vi "Write Identifier Tag.vi"(9 "Array":T3(array[cluster]), 10 "Cluster":T5 {"Main Config"."PR Module Configs"."Settings"."PID 2 Parameters"."output range"."output low" format="%.2f"; "Main Config"."PR Module Configs"."Settings"."PID 2 Parameters"."output range"."output high" min=0.0 max=100.0 format="%.2f"; "Main Config"."PR Module Configs"."Settings"."PID 2 Parameters"."PID gains"."derivative time (Td, min)" format="%.3f"; "Main Config"."PR Module Configs"."Settings"."PID 2 Parameters"."PID gains"."integral time (Ti, min)" format="%.3f"; "Main Config"."PR Module Configs"."Settings"."PID 2 Parameters"."PID gains"."proportional gain (Kc)" format="%.3f"; "Main Config"."Steps"."Control" items=["Pump %", "Setpoint"]; "Main Config"."TCU Module Configs"."Settings"."Huber Unistat 410 Settings"."Address" min=0 max=99 format="%02.0f"; "Main Config"."TCU Module Configs"."Settings"."Julabo FP-50 Settings"."Pump Power" min=0 max=8 step=1; "Main Config"."TCU Module Configs"."Settings"."Lauda Settings"."Pump Power" min=0 max=8 step=1; "Main Config"."Flow Module Configs"."Settings"."Bronkhorst M14 Settings"."Smoothing Steps" min=1 step=1; "Main Config"."Flow Module Configs"."Settings"."Bronkhorst M13 Settings"."Smoothing Steps" min=1 step=1; "Main Config"."Pump Module Configs"."Settings"."Ismatech 3 Channel Settings"."Channel Number" min=0 max=3; "Main Config"."Pump Module Configs"."Settings"."Ismatech 3 Channel Settings"."Pump Number" min=1; "Main Config"."Pump Module Configs"."Settings"."ASIA Pump C"."channel" min=0 max=1 step=1; "Main Config"."Pump Module Configs"."Settings"."Masterflex"."Pump Number" min=1.0 max=20.0 step=1.0; "Main Config"."Pump Module Configs"."Settings"."Ismatech"."Pump Number" min=1.0 max=20.0 step=1.0; "Main Config"."Feed Module Configs"."Settings"."Bronkhorst M14 Settings"."Smoothing Steps" min=1 step=1; "Main Config"."Feed Module Configs"."Settings"."Ismatech 3 Channel Settings"."Channel Number" min=0 max=3; "Main Config"."Feed Module Configs"."Settings"."Ismatech 3 Channel Settings"."Pump Number" min=1; "Main Config"."Feed Module Configs"."Settings"."PID range"."PID Low" min=0.0 max=100.0 format="%.2f"; "Main Config"."Feed Module Configs"."Settings"."PID range"."PID High" format="%.2f"; "Main Config"."Feed Module Configs"."Settings"."PID 2 Parameters"."PID gains"."derivative time (Td, min)" format="%.3f"; "Main Config"."Feed Module Configs"."Settings"."PID 2 Parameters"."PID gains"."integral time (Ti, min)" format="%.3f"; "Main Config"."Feed Module Configs"."Settings"."PID 2 Parameters"."PID gains"."proportional gain (Kc)" format="%.3f"; "Main Config"."Feed Module Configs"."Settings"."Bronkhorst M13 Flow Meter"."Smoothing Steps" min=1 step=1; "Main Config"."Feed Module Configs"."Settings"."ASIA Pump C"."channel" min=0 max=1 step=1; "Main Config"."Feed Module Configs"."Settings"."Ismatech"."Pump Number" min=1.0 max=20.0 step=1.0; "Main Config"."Feed Module Configs"."Settings"."Masterflex"."Pump Number" min=1.0 max=20.0 step=1.0}, 11 "Refnum in":T4) -> ()   [LabVIEW 2018]
uses:
  Drag and Drop/State Cluster.ctl
  support/Message Queue/Message Cluster.ctl
  Drag and Drop/Thumbnail Cluster.ctl
  Drag and Drop/Object Cluster.ctl
  <vilib>/Utility/miscctls.llb/LVRectTypeDef.ctl
  Drag and Drop/Object Type Enum.ctl
  <vilib>/Utility/miscctls.llb/LVPositionTypeDef.ctl
  Config Module/Controls/Main Config Cluster.ctl
  OPC Module Config.ctl
  Scale Module Folder/Measure Instrument/State Enum.ctl
  <vilib>/Utility/miscctls.llb/LVPoint32TypeDef.ctl
  OPC Settings.ctl
  Variable Data Cluster.ctl
  <vilib>/OPCUA/controls/NodeId.ctl
  <vilib>/OPCUA/controls/OPC UA StatusCode.ctl
  <vilib>/OPCUA/controls/Subscription ID.ctl
  <vilib>/OPCUA/controls/OPC UA Client Refnum.ctl
  <vilib>/OPCUA/controls/Subscription Data Change.ctl
  <vilib>/OPCUA/controls/Data Type.ctl
  OPC Tag Data.ctl
  Feed Module/Controls/Feed Module Config Cluster.ctl
  Feed Module/Controls/Feed Module Settings Cluster.ctl
  Ismatec ISM 831C/Controls/Ismatech ISM831C Settings Cluster.ctl
  Masterflex 7550-30/Controls/Settings Cluster.ctl
  Mettler Toledo/Controls/Settings Cluster.ctl
  Bronkhorst M13 Flow Meter/Settings Cluster.ctl
  Measure Instrument/PID 2 Parameters Cluster.ctl
  Measure Instrument/PID Input Enum.ctl
  Measure Instrument/PID 2 Output Enum.ctl
  Tacmina QI/Tacmina QI DAQ Setting.ctl
  KNF Pump/Settings Cluster plus SIMDOS.ctl
  ASIA Pump/Pump Settings.ctl
  VICI M50 Party Mode/Settings Cluster.ctl
  FLOM Pump/Settings Cluster.ctl
  SSI PR Class/SSI PR or LD Settings Cluster.ctl
  Masterflex 75211/Masterflex 75211 DAQ Setting.ctl
  SSI PR Class/SSI P40 Settings Cluster.ctl
  Ismatec 78001/Ismatec 4083.ctl
  Bronkhorst M14 Flow Meter/Settings Cluster.ctl
  Tag VIs/Numeric Alarm Settings Cluster.ctl
  TT Module/Controls/TT Module Config Cluster.ctl
  Acquisition/Hardware Configuration.ctl
  Acquisition/Task Cluster.ctl
  PT Module/Controls/PT Module Config Cluster.ctl
  Scale Module Folder/Feed Module/Controls/Scale Module Config Cluster.ctl
  Scale Module Folder/Feed Module/Controls/Scale Module Settings Cluster.ctl
  Pump Module Folder/Pump Module Config Cluster.ctl
  Pump Module Folder/Pump Module Settings Cluster.ctl
  LabJack Module/Controls/U3 Module Config Cluster.ctl
  Decoration Module/Decoration Module Config Cluster.ctl
  Flow Module Folder/Feed Module/Controls/Flow Module Config Cluster.ctl
  Flow Module Folder/Feed Module/Controls/Flow Module Settings Cluster.ctl
  TCU Module/TCU Module Folder/TCU Module Config Cluster.ctl
  TCU Module/TCU Module Folder/TCU Module Settings Cluster.ctl
  TCU Module/TCU Module Folder/Measure Instrument/Output Devices.ctl
  Huber TCU/Huber Settings.ctl
  Lauda Integral XT-150 TCU/Lauda Settings.ctl
  Julabo Type 1 TCU/Julabo Type 1 TCU Folder/Julabo FP-50 Settings.ctl
  Huber Unistat 410 TCU/Huber Unistat 410 RS485 Settings.ctl
  D-O Module Folder/Not Sure Where this is Used.ctl
  Sequencing/Squence Control.ctl
  D-O Module Folder/D-O Module Config Cluster.ctl
  D-O Module Folder/Valve Clusters.ctl
  D-O Module Folder/D-O Module Settings Cluster.ctl
  D-O Module Folder/D-O Device Settings Cluster.ctl
  VICI Electronic Actuator/VICI Electronic Actuator Settings.ctl
  Pressure Regulator Control Module/Pressure Regulator/Controls/4-20mA Module Config Cluster.ctl
  Pressure Regulator Control Module/Pressure Regulator/Controls/4-20mA Module Settings Cluster.ctl
  Pressure Transmitter/Pressure Transmitter Device Settings.ctl
  Pressure Reg Module/Pressure Regulator Device Settings.ctl
  Sonicator Module Folder/Feed Module/Controls/Sonicator Module Config Cluster.ctl
  Sonicator Module Folder/Feed Module/Controls/Sonicator Module Settings Cluster.ctl
  Sonic Systems P100/Sonic Systems P100 Settings.ctl
  Agitator Module Folder/Feed Module/Controls/Agitator Module Config Cluster.ctl
  Agitator Module Folder/Feed Module/Controls/Agitator Module Settings Cluster.ctl
  IKA EUROSTAR/IKA EUROSTAR Settings.ctl
  Centrifuge Module Folder/Centrifuge Module Config Cluster.ctl
  Centrifuge Module Folder/Centrifuge Module Settings Cluster.ctl
  EPOS4/Controls/Device Selection.ctl
  EPOS4/Controls/EPOS Communication Settings.ctl
  <vilib>/OPCUA/controls/OPC UA Server Refnum.ctl
  <vilib>/OPCUA/controls/OPC UA Variable Node Refnum.ctl
  <vilib>/OPCUA/server/Write String.vi
  <vilib>/OPCUA/NI OPC UA Server.lvlib
  support/Message Queue/Message Queue.lvlib
  TT Module/TT Module.lvlib
  Masterflex 75211/Masterflex 75211.lvlib
  Masterflex 7550-30/Masterflex 7550-30.lvlib
  Ismatec ISM 831C/Ismatec ISM 831C.lvlib
  Tacmina QI/Tacmina QI.lvlib
  KNF Pump/KNF SIMDOS.lvlib
  VICI M50 Party Mode/VICI M6 M50 Party Mode.lvlib
  FLOM Pump/FLOM Pump.lvlib
  ASIA Pump.lvlib
  Mettler Toledo/Mettler Toledo.lvlib
  Bronkhorst M13 Flow Meter/Bronkhorst M13 Flow Meter.lvlib
  SSI PR Class/SSI PR or LD Pump.lvlib
  SSI PR Class/SSI P40 Pump.lvlib
  Ismatec 78001/Ismatec 4308.lvlib
  Bronkhorst M14 Flow Meter/Bronkhorst M14 Flow Meter.lvlib
  Feed Module/Feed Module.lvlib
  DAQ/DAQ.lvlib
  PT Module/PT Module.lvlib
  Scale Module Folder/Scale Module.lvlib
  Pump Module Folder/Pump Module.lvlib
  LabJack Module/U3 Module.lvlib
  Flow Module Folder/Flow Module.lvlib
  Huber TCU/Huber Ministat 230 TCU.lvlib
  Lauda Integral XT-150 TCU/Lauda TCU.lvlib
  Julabo Type 1 TCU/Julabo Type 1 TCU Folder/Julabo Type FP-50 TCU.lvlib
  Huber Unistat 410 TCU/Huber Unistat 410 TCU.lvlib
  TCU Module/TCU Module Folder/TCU Module.lvlib
  Sequencing/Sequencing Library.lvlib
  D-O Module Folder/D-O Module.lvlib
  D-O Module Folder/DIO Valve/VICI Electronic Actuator.lvlib
  Pressure Transmitter/Pressure Transmitter Library.lvlib
  Pressure Reg Module/Pressure Regulator Library.lvlib
  Pressure Regulator Control Module/Pressure Regulator/4-20mA Module.lvlib
  OPC UA.lvlib
  Scale Module Folder/Measure Instrument/Scale Module Engine.lvlib
  Sonic Systems P100/Sonic Systems P100.lvlib
  Sonicator Module Folder/Sonicator Module.lvlib
  Agitator Module Folder/Agitator Module.lvlib
  Config Module/Config Module.lvlib
  Drag and Drop/Drag and Drop.lvlib
  EPOS4/EPOS4.lvlib
  Centrifuge Module Folder/Centrifuge Module.lvlib
  IKA EUROSTAR/IKA EUROSTAR.lvlib
panel:
  # "Agitator Settings"
  # "Sonicator Settings"
  # "Instrument Settings"
  # "Instrument Settings"
  # "Output Instruments"
  # "Flow Meter Settings"
  # "Output Instruments"
  # "Scale Settings"
  # "Output Instruments"
  # "Input Instruments"
types:
  T1 = typedef "NodeId.ctl" = string
  T2 = typedef "OPC UA Variable Node Refnum.ctl" = refnum<k21>
  T3 = cluster{"property node ID":T1, "OPC UA variable node refnum out":T2, "name":string}[]
  T4 = typedef "OPC UA Server Refnum.ctl" = refnum<k21>
  T5 = typedef "Drag and Drop.lvlib/State Cluster.ctl" = cluster{"VI refs":refnum<vi>[], "Queues":refnum<queue>[], "[Thumbnails]":T6[], "Drag Object Idx":i32, "[Objects]":T7[], "Active Object":i32, "Drop Offset":T10, "Process Name":string, "Main Config":T11, "Campaign Filepath":path, "Config Changed?":bool}
  T6 = typedef "Thumbnail Cluster.ctl" = cluster{"Path":path, "Rectangle":cluster{"left":i16, "top":i16, "right":i16, "bottom":i16}}
  T7 = typedef "Object Cluster.ctl" = cluster{"BMP Path":path, "Anchor Position":cluster{"X":i32, "Y":i32}, "Hot Spot":T8, "Type":T9, "Parameters":variant}
  T8 = typedef "LVRectTypeDef.ctl" = cluster{"Left":i16, "Top":i16, "Right":i16, "Bottom":i16}
  T9 = typedef "Object Type Enum.ctl" = enum16{"Icon", "Line", "Text", "Feed Module"}
  T10 = typedef "LVPositionTypeDef.ctl" = cluster{"Left":i32, "Top":i32}
  T11 = typedef "Config Module.lvlib/Main Config Cluster.ctl" = cluster{"Notebook":string, "OPC Module Configs":T12[], "Feed Module Configs":T21[], "Log File Path":path, "TT Module Configs":T41[], "DAQ Config":T42, "PT Module Configs":T44[], "Scale Module Configs":T45[], "Pump Module Configs":T47[], "U3 Module Configs":T49[], "Decoration Module Configs":T50[], "Flow Module Configs":T51[], "TCU Module Configs":T53[], "Steps":T60, "Abort":bool, "DO Module Configs":T62[], "PR Module Configs":T67[], "SC Module Configs":T71[], "AM Module Configs":T74[], "CM Module Configs":T77[], "Cycle Period":dbl}
  T12 = typedef "OPC UA.lvlib/OPC Module Config.ctl" = cluster{"State":T13, "GUID":string, "Process Name":string, "User name":string, "Drop Coords":T14, "Configuration":T15, "First Iteration":bool, "Data":cluster{"Object Name":string, "Variable Array":T16[]}[], "Load Count":i32, "Log Started":bool, "subscription ID out":T18, "OPC UA client refnum out":T19, "Event Registration Refnum":refnum<event-registration>, "Start Time":timestamp, "Current Time":timestamp, "Tag Data":T20[]}
  T13 = typedef "Scale Module.lvlib/Scale Module Engine.lvlib/State Enum.ctl" = enum16{"Measuring", "Idle"}
  T14 = typedef "LVPoint32TypeDef.ctl" = cluster{"Horizontal":i32, "Vertical":i32}
  T15 = typedef "OPC UA.lvlib/OPC Settings.ctl" = cluster{"Cycle Period":dbl, "server endpoint URL":string, "security policy":cluster{"message mode":enum16{"None", "Sign", "Sign and Encrypt"}, "security":enum16{"Basic256", "Basic128Rsa15"}}, "Trust Any Server":bool}
  T16 = typedef "OPC UA.lvlib/Variable Data Cluster.ctl" = cluster{"node ID":T1, "browse name":string, "status":T17, "timestamp":timestamp, "value ":variant}
  T17 = typedef "OPC UA StatusCode.ctl" = u32
  T18 = typedef "Subscription ID.ctl" = u32
  T19 = typedef "OPC UA Client Refnum.ctl" = refnum<k21>
  T20 = typedef "OPC UA.lvlib/OPC Tag Data.ctl" = cluster{"Include this Device":bool, "Device Name":string, "OPC Tag Data":cluster{"Tag":string, "Value":variant, "Time Stamp":timestamp}[]}
  T21 = typedef "Feed Module.lvlib/Feed Module Config Cluster.ctl" = cluster{"GUID":string, "Drop Coords":T14, "Process Name":string, "User name":string, "Queue Name":string, "Settings":T22, "Settings Load Count":i32, "OP Load Count":i32}
  T22 = typedef "Feed Module.lvlib/Feed Module Settings Cluster.ctl" = cluster{"Cycle Period":dbl, "Ismatech":T23, "Masterflex":T24, "Mettler":T25, "Bronkhorst M13 Flow Meter":T26, "PID 2 Parameters":T27, "Manual Entry":dbl, "Auto?":bool, "PID range":cluster{"PID High":dbl, "PID Low":dbl, "High Warning":dbl}, "Tacmina Settings":T30, "KNF SIMDOS Settings":T31, "ASIA Pump C":T32, "VICI Settings":T33, "FLOM Settings":T34, "SSI PR/LD Settings":T35, "Masterflex 75211 Settings":T36, "SSI P40 Settings":T37, "Ismatech 3 Channel Settings":T38, "Bronkhorst M14 Settings":T39, "Reset Totalizer":bool, "Input Num Alarm Settings":T40[], "Control Type":enum32{"g/min", "ml/min"}, "Front End Display Options":cluster{"Temperature":bool, "Scale Grams":bool, "Density":bool, "Flow (g/min)":bool, "Flow (ml/min)":bool, "PSIG":bool, "Total Grams":bool, "Updated":bool}}
  T23 = typedef "Ismatec ISM 831C.lvlib/Ismatech ISM831C Settings Cluster.ctl" = cluster{"VISA resource name":refnum<visa-resource-name>, "Simulated?":bool, "Pump Number":dbl, "Reverse?":bool}
  T24 = typedef "Masterflex 7550-30.lvlib/Settings Cluster.ctl" = cluster{"VISA resource name":refnum<visa-resource-name>, "Simulated?":bool, "Pump Number":dbl, "Reverse?":bool}
  T25 = typedef "Mettler Toledo.lvlib/Settings Cluster.ctl" = cluster{"VISA resource name":refnum<visa-resource-name>, "Simulated?":bool}
  T26 = typedef "Bronkhorst M13 Flow Meter.lvlib/Settings Cluster.ctl" = cluster{"VISA resource name":refnum<visa-resource-name>, "Simulated?":bool, "Smoothing Steps":i32}
  T27 = typedef "PID 2 Parameters Cluster.ctl" = cluster{"Input Device":T28, "Output Device":T29, "Setpoint":dbl, "PID gains":cluster{"proportional gain (Kc)":dbl, "integral time (Ti, min)":dbl, "derivative time (Td, min)":dbl}}
  T28 = typedef "PID Input Enum.ctl" = enum16{"Default", "Bronkhorst M13", "Bronkhorst M14", "Scale Rate of Change"}
  T29 = typedef "PID 2 Output Enum.ctl" = enum16{"Default", "Ismatec ISM 4308", "Ismatec ISM 831C", "Masterflex 7550-30", "VICI M6", "VICI M50", "Tacmina QI", "KNF SIMDOS", "ASIA Type C", "FLOM UI-22-11", "SSI PR/LD", "SSI P40", "Masterflex 75211-70"}
  T30 = typedef "Tacmina QI.lvlib/Tacmina QI DAQ Setting.ctl" = cluster{"Analog DAQ Task":refnum<k21>, "Digital DAQ Task":refnum<k21>}
  T31 = typedef "KNF SIMDOS.lvlib/Settings Cluster plus SIMDOS.ctl" = cluster{"VISA resource name":refnum<visa-resource-name>, "Simulated?":bool}
  T32 = typedef "ASIA Pump.lvlib/Pump Settings.ctl" = cluster{"ASIA Pump #":i32, "channel":i32, "Simulated":bool}
  T33 = typedef "VICI M6 M50 Party Mode.lvlib/Settings Cluster.ctl" = cluster{"VISA resource name":refnum<visa-resource-name>, "Pump ID":string, "Pump Head Vol":dbl, "Reverse?":bool, "Simulated?":bool}
  T34 = typedef "FLOM Pump.lvlib/Settings Cluster.ctl" = cluster{"VISA resource name":refnum<visa-resource-name>, "Simulated?":bool, "Pump Number":dbl}
  T35 = typedef "SSI PR or LD Pump.lvlib/SSI PR or LD Settings Cluster.ctl" = cluster{"VISA resource name":refnum<visa-resource-name>, "Simulated?":bool}
  T36 = typedef "Masterflex 75211.lvlib/Masterflex 75211 DAQ Setting.ctl" = cluster{"Analog DAQ Task":refnum<k21>, "Digital DAQ Task":refnum<k21>}
  T37 = typedef "SSI P40 Pump.lvlib/SSI P40 Settings Cluster.ctl" = cluster{"VISA resource name":refnum<visa-resource-name>, "Simulated?":bool}
  T38 = typedef "Ismatec 4308.lvlib/Ismatec 4083.ctl" = cluster{"VISA resource name":refnum<visa-resource-name>, "Pump Number":i16, "Channel Number":i16, "Simulated?":bool, "Reverse?":bool}
  T39 = typedef "Bronkhorst M14 Flow Meter.lvlib/Settings Cluster.ctl" = cluster{"VISA resource name":refnum<visa-resource-name>, "Simulated?":bool, "Smoothing Steps":i32}
  T40 = typedef "Numeric Alarm Settings Cluster.ctl" = cluster{"enable? (F)":bool, "name":string, "alarm type":enum16{"HI_HI", "HI", "LO", "LO_LO"}, "level/change":dbl, "deadband/time":dbl, "alarm delay":dbl, "priority":u32, "ack type":enum16{"Auto", "User", "None", "Each Occurrence"}, "area":string, "description":string, "log? (T)":bool}
  T41 = typedef "TT Module.lvlib/TT Module Config Cluster.ctl" = cluster{"GUID":string, "Drop Coords":T14, "Input Channel Tag Name ":string, "Process Name":string, "User name":string, "Queue Name":string, "Input Channel Numeric Alarm Settings":T40[]}
  T42 = typedef "DAQ.lvlib/Hardware Configuration.ctl" = cluster{"Tasks Array":T43[]}
  T43 = typedef "Task Cluster.ctl" = cluster{"DAQmx Task":refnum<k21>, "Read-Write Radio":enum32{"Read", "Write"}}
  T44 = typedef "PT Module.lvlib/PT Module Config Cluster.ctl" = cluster{"GUID":string, "Drop Coords":T14, "Input Channel Tag Name ":string, "Process Name":string, "User name":string, "Queue Name":string, "Input Channel Numeric Alarm Settings":T40[]}
  T45 = typedef "Scale Module.lvlib/Scale Module Config Cluster.ctl" = cluster{"GUID":string, "Drop Coords":T14, "Process Name":string, "User name":string, "Queue Name":string, "Settings":T46, "Load Count":i32}
  T46 = typedef "Scale Module.lvlib/Scale Module Settings Cluster.ctl" = cluster{"Cycle Period":dbl, "Mettler":T25, "Scale Type":string}
  T47 = typedef "Pump Module.lvlib/Pump Module Config Cluster.ctl" = cluster{"GUID":string, "Drop Coords":T14, "Process Name":string, "User name":string, "Queue Name":string, "Settings":T48, "Load Count":i32}
  T48 = typedef "Pump Module.lvlib/Pump Module Settings Cluster.ctl" = cluster{"Cycle Period":dbl, "Manual Entry":dbl, "Output Device":T29, "Ismatech":T23, "Ismatech 3 Channel Settings":T38, "Masterflex":T24, "VICI Settings":T33, "Tacmina Settings":T30, "KNF SIMDOS Settings":T31, "ASIA Pump C":T32, "FLOM Settings":T34, "SSI PR/LD Settings":T35, "SSI P40 Settings":T35, "Masterflex 75211 Settings":T36, "Pump Calibration File":path, "Calibration Slope":dbl, "Calibration Y Intercept":dbl, "Pump Cal Enum":u16, "Reset Totalizer":bool}
  T49 = typedef "U3 Module.lvlib/U3 Module Config Cluster.ctl" = cluster{"GUID":string, "Drop Coords":T14, "AI Channel Number":enum16{"Default", "AI0", "AI1", "AI2", "AI3", "AI4", "AI5", "AI6", "AI7"}, "Process Name":string, "User name":string, "Queue Name":string, "Input Channel Numeric Alarm Settings":T40[]}
  T50 = typedef "Decoration Module Config Cluster.ctl" = cluster{"GUID":string, "Drop Coords":T14, "Decoration Filepath":path}
  T51 = typedef "Flow Module.lvlib/Flow Module Config Cluster.ctl" = cluster{"GUID":string, "Drop Coords":T14, "Process Name":string, "User name":string, "Queue Name":string, "Settings":T52, "Load Count":i32}
  T52 = typedef "Flow Module.lvlib/Flow Module Settings Cluster.ctl" = cluster{"Cycle Period":dbl, "Flow Meter Type":string, "Bronkhorst M13 Settings":T26, "Bronkhorst M14 Settings":T39, "Reset Totalizer":bool}
  T53 = typedef "TCU Module.lvlib/TCU Module Config Cluster.ctl" = cluster{"GUID":string, "Drop Coords":T14, "Process Name":string, "User name":string, "Queue Name":string, "Settings":T54, "Load Count":i32, "Power Level Changed":bool}
  T54 = typedef "TCU Module.lvlib/TCU Module Settings Cluster.ctl" = cluster{"Cycle Period":dbl, "Setpoint Entry":dbl, "Output Device":T55, "Huber Ministat 230 Settings":T56, "Lauda Settings":T57, "Julabo FP-50 Settings":T58, "Internal Control?":bool, "Huber Unistat 410 Settings":T59}
  T55 = typedef "Output Devices.ctl" = enum16{"Default", "Huber Ministat 230", "Huber Unistat 410", "Lauda XT-150", "Julabo FP-50"}
  T56 = typedef "Huber Ministat 230 TCU.lvlib/Huber Settings.ctl" = cluster{"VISA resource name":refnum<visa-resource-name>, "Simulated?":bool}
  T57 = typedef "Lauda TCU.lvlib/Lauda Settings.ctl" = cluster{"VISA resource name":refnum<visa-resource-name>, "Simulated?":bool, "Pump Power":i32}
  T58 = typedef "Julabo Type FP-50 TCU.lvlib/Julabo FP-50 Settings.ctl" = cluster{"VISA resource name":refnum<visa-resource-name>, "Simulated?":bool, "Pump Power":i32}
  T59 = typedef "Huber Unistat 410 TCU.lvlib/Huber Unistat 410 RS485 Settings.ctl" = cluster{"VISA resource name":refnum<visa-resource-name>, "Address":i8, "Simulated?":bool}
  T60 = typedef "Not Sure Where this is Used.ctl" = T61[]
  T61 = typedef "Sequencing Library.lvlib/Squence Control.ctl" = cluster{"Module":string, "Control":u16, "Value":dbl, "Wait (sec)":dbl}
  T62 = typedef "D-O Module.lvlib/D-O Module Config Cluster.ctl" = cluster{"GUID":string, "Drop Coords":T14, "Process Name":string, "User name":string, "Queue Name":string, "Settings":T63, "Load Count":i32}
  T63 = typedef "D-O Module.lvlib/Valve Clusters.ctl" = cluster{"Valve Settings":T64, "Valve Type":enum16{"Default", "Digital Output Valve", "VICI Electronic Actuator"}, "Time On (Sec)":dbl, "Time Off (Sec)":dbl, "Run?":bool}
  T64 = typedef "D-O Module.lvlib/D-O Module Settings Cluster.ctl" = cluster{"D-O Settings":T65, "VICI Electronic Actuator":T66}
  T65 = typedef "D-O Module.lvlib/D-O Device Settings Cluster.ctl" = cluster{"DAQmx Task Name":refnum<k21>, "Output Channel":u16, "Output Channel Names":string[]}
  T66 = typedef "VICI Electronic Actuator.lvlib/VICI Electronic Actuator Settings.ctl" = cluster{"VISA resource name":refnum<visa-resource-name>, "Mode":enum16{"Two Positions With Stops", "Two Positions Without Stops", "Mutiposition"}, "Simulated":bool}
  T67 = typedef "4-20mA Module.lvlib/4-20mA Module Config Cluster.ctl" = cluster{"GUID":string, "Drop Coords":T14, "Process Name":string, "User name":string, "Queue Name":string, "Settings":T68, "Settings Load Count":i32}
  T68 = typedef "4-20mA Module.lvlib/4-20mA Module Settings Cluster.ctl" = cluster{"Cycle Period":dbl, "PID 2 Parameters":cluster{"Input Device":enum16{"Default", "4-20mA"}, "Output Device":enum16{"Default", "Equilibar Pressure Reg", "Flow Regulator"}, "Setpoint":dbl, "PID gains":cluster{"proportional gain (Kc)":dbl, "integral time (Ti, min)":dbl, "derivative time (Td, min)":dbl}, "output range":cluster{"output low":dbl, "output high":dbl}}, "Manual Entry":dbl, "Auto?":bool, "4-20mA Input Settings":T69, "4-20mA Out Settings":T70, "Input Channel Tag Name ":string}
  T69 = typedef "Pressure Transmitter Library.lvlib/Pressure Transmitter Device Settings.ctl" = cluster{"Input Channel ":u16}
  T70 = typedef "Pressure Regulator Library.lvlib/Pressure Regulator Device Settings.ctl" = cluster{"Output DAQ Task":refnum<k21>}
  T71 = typedef "Sonicator Module.lvlib/Sonicator Module Config Cluster.ctl" = cluster{"GUID":string, "Drop Coords":T14, "Process Name":string, "User name":string, "Queue Name":string, "Settings":T72, "Load Count":i32}
  T72 = typedef "Sonicator Module.lvlib/Sonicator Module Settings Cluster.ctl" = cluster{"Cycle Period":dbl, "Sonicator Type":string, "SS P100 Settings":T73, "Setpoint (µm)":dbl, "Cutoff (W)":dbl}
  T73 = typedef "Sonic Systems P100.lvlib/Sonic Systems P100 Settings.ctl" = cluster{"VISA resource name":refnum<visa-resource-name>, "Simulated?":bool}
  T74 = typedef "Agitator Module.lvlib/Agitator Module Config Cluster.ctl" = cluster{"GUID":string, "Drop Coords":T14, "Process Name":string, "User name":string, "Queue Name":string, "Settings":T75, "Load Count":i32}
  T75 = typedef "Agitator Module.lvlib/Agitator Module Settings Cluster.ctl" = cluster{"Cycle Period":dbl, "Agitator Type":string, "Setpoint (µm)":dbl, "IKA EUROSTAR Settings":T76}
  T76 = typedef "IKA EUROSTAR.lvlib/IKA EUROSTAR Settings.ctl" = cluster{"VISA resource name":refnum<visa-resource-name>, "Simulated?":bool}
  T77 = typedef "Centrifuge Module.lvlib/Centrifuge Module Config Cluster.ctl" = cluster{"GUID":string, "Drop Coords":T14, "Process Name":string, "User name":string, "Queue Name":string, "Settings":T78, "Load Count":i32}
  T78 = typedef "Centrifuge Module.lvlib/Centrifuge Module Settings Cluster.ctl" = cluster{"Cycle Period":dbl, "Manual Entry":dbl, "Output Device":T79, "EPOS4 Settings":T80}
  T79 = typedef "Device Selection.ctl" = enum16{"Default", "EPOS4"}
  T80 = typedef "EPOS4.lvlib/EPOS Communication Settings.ctl" = cluster{"VISA resource name":refnum<visa-resource-name>, "axis":cluster{"keyHandle":u32, "nodeId":u16}, "Simulated?":bool}
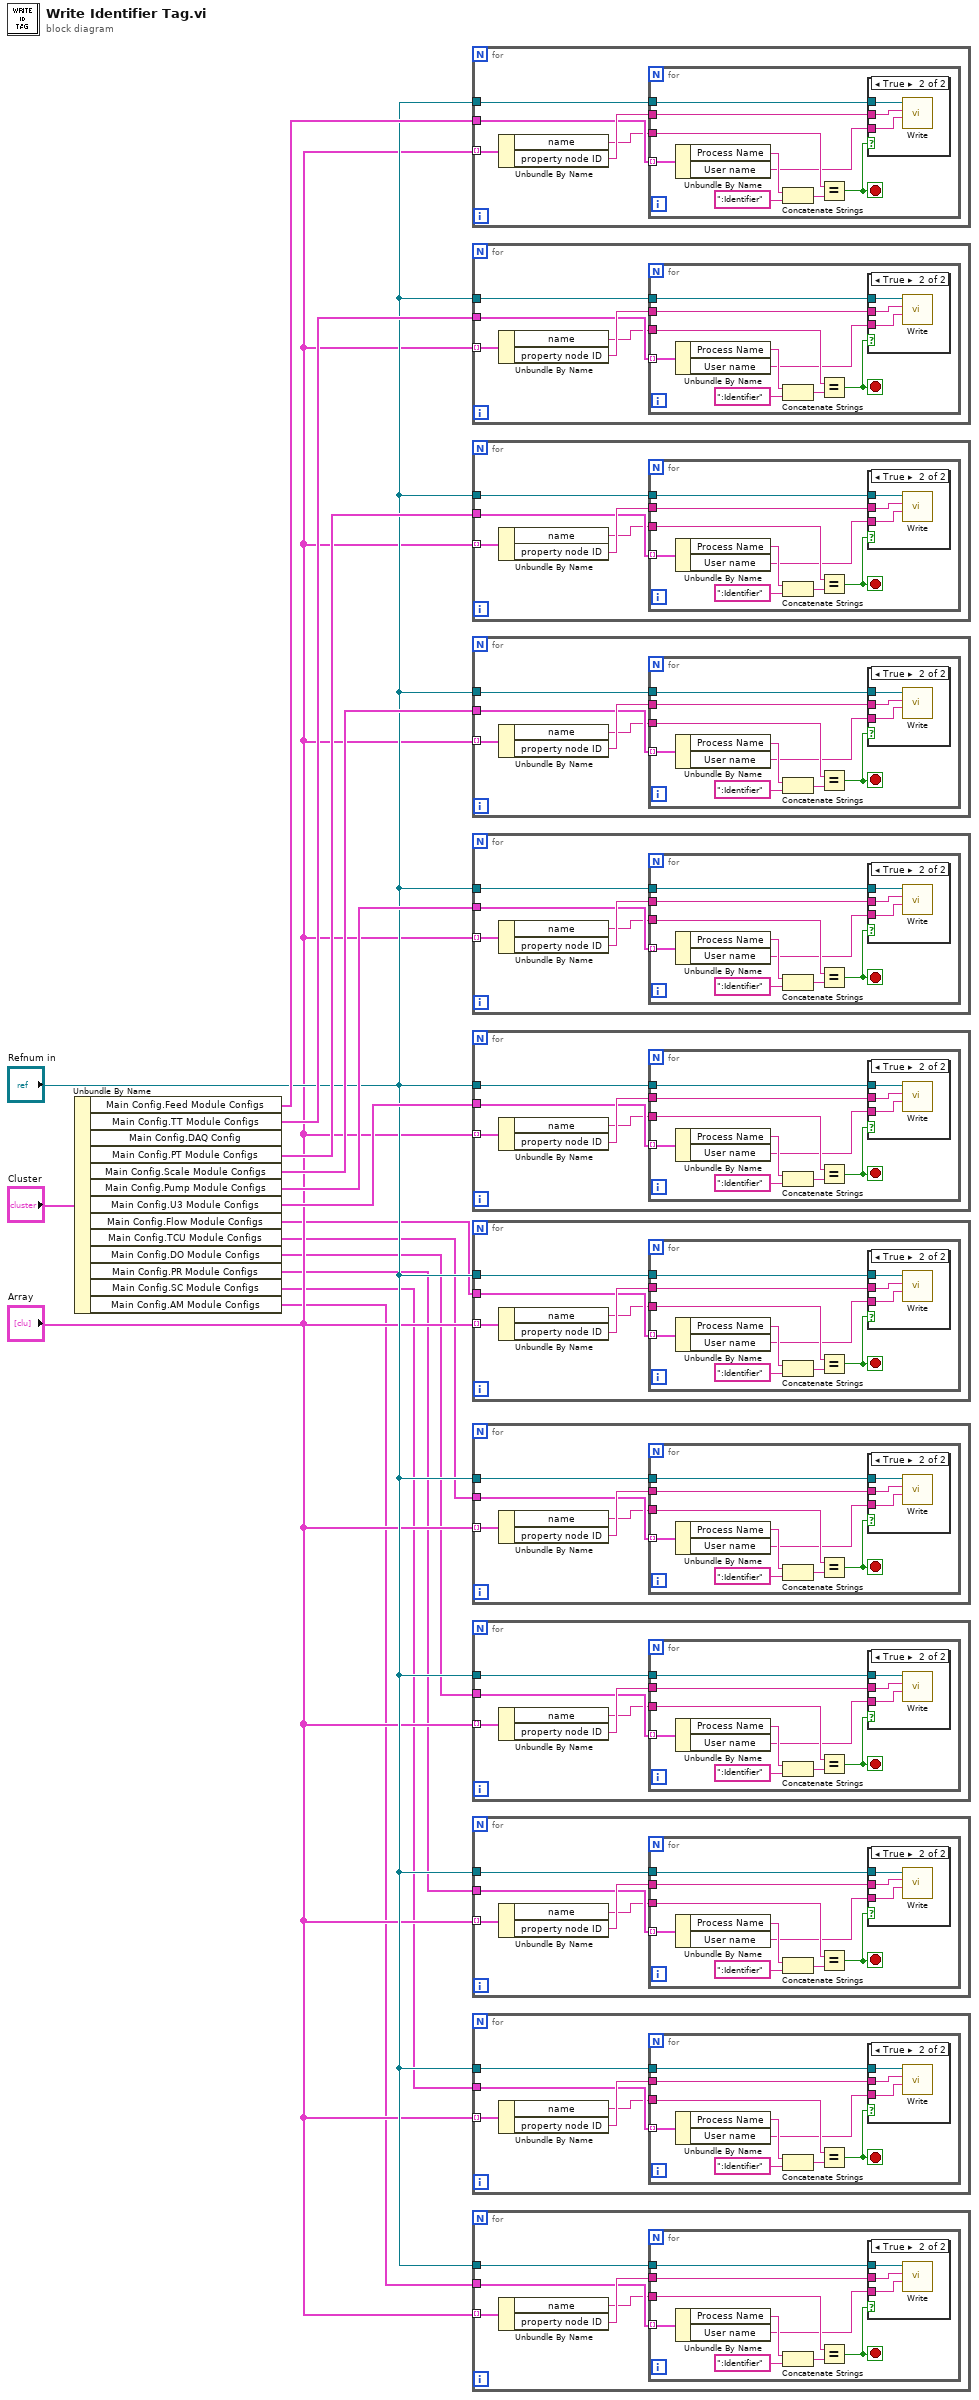
[diagram p0: block diagram]
diagram:
  n1 = Unbundle By Name("Cluster") -> ("Main Config.Feed Module Configs"=w14:T21[], "Main Config.TT Module Configs"=w13:T41[], "Main Config.PT Module Configs"=w12:T44[], "Main Config.Scale Module Configs"=w11:T45[], "Main Config.Pump Module Configs"=w10:T47[], "Main Config.U3 Module Configs"=w9:T49[], "Main Config.Flow Module Configs"=w6:T51[], "Main Config.TCU Module Configs"=w5:T53[], "Main Config.DO Module Configs"=w4:T62[], "Main Config.PR Module Configs"=w3:T67[], "Main Config.SC Module Configs"=w2:T71[], "Main Config.AM Module Configs"=w1:T74[])  [unwired: 1 out]
  n2 = for {
    tunnel: "Array" -> [w20] mode=indexing
    tunnel: "Refnum in" -> [w18]
    tunnel: w14 -> [w17]
    n3 = Unbundle By Name(w20) -> ("name"=w16:string, "property node ID"=w19:T1)
    n4 = for {
      tunnel: w19 -> [w29]
      tunnel: w18 -> [w28]
      tunnel: w17 -> [w27] mode=indexing
      tunnel: w16 -> [w26]
      stop <- w21 stop-if-true
      n5 = Unbundle By Name(w27) -> ("Process Name"=w25:string, "User name"=w22:string)
      n6 = Concatenate Strings(w25, ":Identifier" ("string")) -> (w23:string)
      n7 = Equal?(x=w26, y=w23) -> (x = y?=w21:bool)
      n8 = case shown="True" w21 {
        tunnel: w29 -> [_ w32]
        tunnel: w28 -> [_ w31]
        tunnel: w22 -> [_ w30]
        frame False {
        }
        frame True {
          n9 = call-poly <vilib>:"Write.vi"("value"=w30, "node ID"=w32, "OPC UA server refnum in"=w31) -> ()  [unwired: 6 in, 3 out]
        }
      }
    }
  }
  n10 = for {
    tunnel: "Array" -> [w37] mode=indexing
    tunnel: "Refnum in" -> [w35]
    tunnel: w13 -> [w34]
    n11 = Unbundle By Name(w37) -> ("name"=w33:string, "property node ID"=w36:T1)
    n12 = for {
      tunnel: w36 -> [w46]
      tunnel: w35 -> [w45]
      tunnel: w34 -> [w44] mode=indexing
      tunnel: w33 -> [w43]
      stop <- w38 stop-if-true
      n13 = Unbundle By Name(w44) -> ("Process Name"=w42:string, "User name"=w39:string)
      n14 = Concatenate Strings(w42, ":Identifier" ("string")) -> (w40:string)
      n15 = Equal?(x=w43, y=w40) -> (x = y?=w38:bool)
      n16 = case shown="True" w38 {
        tunnel: w46 -> [_ w49]
        tunnel: w45 -> [_ w48]
        tunnel: w39 -> [_ w47]
        frame False {
        }
        frame True {
          n17 = call-poly <vilib>:"Write.vi"("value"=w47, "node ID"=w49, "OPC UA server refnum in"=w48) -> ()  [unwired: 6 in, 3 out]
        }
      }
    }
  }
  n18 = for {
    tunnel: "Array" -> [w54] mode=indexing
    tunnel: "Refnum in" -> [w52]
    tunnel: w12 -> [w51]
    n19 = Unbundle By Name(w54) -> ("name"=w50:string, "property node ID"=w53:T1)
    n20 = for {
      tunnel: w53 -> [w63]
      tunnel: w52 -> [w62]
      tunnel: w51 -> [w61] mode=indexing
      tunnel: w50 -> [w60]
      stop <- w55 stop-if-true
      n21 = Unbundle By Name(w61) -> ("Process Name"=w59:string, "User name"=w56:string)
      n22 = Concatenate Strings(w59, ":Identifier" ("string")) -> (w57:string)
      n23 = Equal?(x=w60, y=w57) -> (x = y?=w55:bool)
      n24 = case shown="True" w55 {
        tunnel: w63 -> [_ w66]
        tunnel: w62 -> [_ w65]
        tunnel: w56 -> [_ w64]
        frame False {
        }
        frame True {
          n25 = call-poly <vilib>:"Write.vi"("value"=w64, "node ID"=w66, "OPC UA server refnum in"=w65) -> ()  [unwired: 6 in, 3 out]
        }
      }
    }
  }
  n26 = for {
    tunnel: "Array" -> [w71] mode=indexing
    tunnel: "Refnum in" -> [w69]
    tunnel: w11 -> [w68]
    n27 = Unbundle By Name(w71) -> ("name"=w67:string, "property node ID"=w70:T1)
    n28 = for {
      tunnel: w70 -> [w80]
      tunnel: w69 -> [w79]
      tunnel: w68 -> [w78] mode=indexing
      tunnel: w67 -> [w77]
      stop <- w72 stop-if-true
      n29 = Unbundle By Name(w78) -> ("Process Name"=w76:string, "User name"=w73:string)
      n30 = Concatenate Strings(w76, ":Identifier" ("string")) -> (w74:string)
      n31 = Equal?(x=w77, y=w74) -> (x = y?=w72:bool)
      n32 = case shown="True" w72 {
        tunnel: w80 -> [_ w83]
        tunnel: w79 -> [_ w82]
        tunnel: w73 -> [_ w81]
        frame False {
        }
        frame True {
          n33 = call-poly <vilib>:"Write.vi"("value"=w81, "node ID"=w83, "OPC UA server refnum in"=w82) -> ()  [unwired: 6 in, 3 out]
        }
      }
    }
  }
  n34 = for {
    tunnel: "Array" -> [w88] mode=indexing
    tunnel: "Refnum in" -> [w86]
    tunnel: w10 -> [w85]
    n35 = Unbundle By Name(w88) -> ("name"=w84:string, "property node ID"=w87:T1)
    n36 = for {
      tunnel: w87 -> [w97]
      tunnel: w86 -> [w96]
      tunnel: w85 -> [w95] mode=indexing
      tunnel: w84 -> [w94]
      stop <- w89 stop-if-true
      n37 = Unbundle By Name(w95) -> ("Process Name"=w93:string, "User name"=w90:string)
      n38 = Concatenate Strings(w93, ":Identifier" ("string")) -> (w91:string)
      n39 = Equal?(x=w94, y=w91) -> (x = y?=w89:bool)
      n40 = case shown="True" w89 {
        tunnel: w97 -> [_ w100]
        tunnel: w96 -> [_ w99]
        tunnel: w90 -> [_ w98]
        frame False {
        }
        frame True {
          n41 = call-poly <vilib>:"Write.vi"("value"=w98, "node ID"=w100, "OPC UA server refnum in"=w99) -> ()  [unwired: 6 in, 3 out]
        }
      }
    }
  }
  n42 = for {
    tunnel: "Array" -> [w105] mode=indexing
    tunnel: w9 -> [w103]
    tunnel: "Refnum in" -> [w101]
    n43 = Unbundle By Name(w105) -> ("name"=w102:string, "property node ID"=w104:T1)
    n44 = for {
      tunnel: w104 -> [w114]
      tunnel: w101 -> [w113]
      tunnel: w103 -> [w112] mode=indexing
      tunnel: w102 -> [w111]
      stop <- w106 stop-if-true
      n45 = Unbundle By Name(w112) -> ("Process Name"=w110:string, "User name"=w107:string)
      n46 = Concatenate Strings(w110, ":Identifier" ("string")) -> (w108:string)
      n47 = Equal?(x=w111, y=w108) -> (x = y?=w106:bool)
      n48 = case shown="True" w106 {
        tunnel: w114 -> [_ w117]
        tunnel: w113 -> [_ w116]
        tunnel: w107 -> [_ w115]
        frame False {
        }
        frame True {
          n49 = call-poly <vilib>:"Write.vi"("value"=w115, "node ID"=w117, "OPC UA server refnum in"=w116) -> ()  [unwired: 6 in, 3 out]
        }
      }
    }
  }
  n50 = for {
    tunnel: "Array" -> [w122] mode=indexing
    tunnel: "Refnum in" -> [w120]
    tunnel: w6 -> [w119]
    n51 = Unbundle By Name(w122) -> ("name"=w118:string, "property node ID"=w121:T1)
    n52 = for {
      tunnel: w121 -> [w131]
      tunnel: w120 -> [w130]
      tunnel: w119 -> [w129] mode=indexing
      tunnel: w118 -> [w128]
      stop <- w123 stop-if-true
      n53 = Unbundle By Name(w129) -> ("Process Name"=w127:string, "User name"=w124:string)
      n54 = Concatenate Strings(w127, ":Identifier" ("string")) -> (w125:string)
      n55 = Equal?(x=w128, y=w125) -> (x = y?=w123:bool)
      n56 = case shown="True" w123 {
        tunnel: w131 -> [_ w134]
        tunnel: w130 -> [_ w133]
        tunnel: w124 -> [_ w132]
        frame False {
        }
        frame True {
          n57 = call-poly <vilib>:"Write.vi"("value"=w132, "node ID"=w134, "OPC UA server refnum in"=w133) -> ()  [unwired: 6 in, 3 out]
        }
      }
    }
  }
  n58 = for {
    tunnel: "Array" -> [w139] mode=indexing
    tunnel: "Refnum in" -> [w137]
    tunnel: w5 -> [w136]
    n59 = Unbundle By Name(w139) -> ("name"=w135:string, "property node ID"=w138:T1)
    n60 = for {
      tunnel: w138 -> [w148]
      tunnel: w137 -> [w147]
      tunnel: w136 -> [w146] mode=indexing
      tunnel: w135 -> [w145]
      stop <- w140 stop-if-true
      n61 = Unbundle By Name(w146) -> ("Process Name"=w144:string, "User name"=w141:string)
      n62 = Concatenate Strings(w144, ":Identifier" ("string")) -> (w142:string)
      n63 = Equal?(x=w145, y=w142) -> (x = y?=w140:bool)
      n64 = case shown="True" w140 {
        tunnel: w148 -> [_ w151]
        tunnel: w147 -> [_ w150]
        tunnel: w141 -> [_ w149]
        frame False {
        }
        frame True {
          n65 = call-poly <vilib>:"Write.vi"("value"=w149, "node ID"=w151, "OPC UA server refnum in"=w150) -> ()  [unwired: 6 in, 3 out]
        }
      }
    }
  }
  n66 = for {
    tunnel: "Array" -> [w156] mode=indexing
    tunnel: "Refnum in" -> [w154]
    tunnel: w4 -> [w153]
    n67 = Unbundle By Name(w156) -> ("name"=w152:string, "property node ID"=w155:T1)
    n68 = for {
      tunnel: w155 -> [w165]
      tunnel: w154 -> [w164]
      tunnel: w153 -> [w163] mode=indexing
      tunnel: w152 -> [w162]
      stop <- w157 stop-if-true
      n69 = Unbundle By Name(w163) -> ("Process Name"=w161:string, "User name"=w158:string)
      n70 = Concatenate Strings(w161, ":Identifier" ("string")) -> (w159:string)
      n71 = Equal?(x=w162, y=w159) -> (x = y?=w157:bool)
      n72 = case shown="True" w157 {
        tunnel: w165 -> [_ w168]
        tunnel: w164 -> [_ w167]
        tunnel: w158 -> [_ w166]
        frame False {
        }
        frame True {
          n73 = call-poly <vilib>:"Write.vi"("value"=w166, "node ID"=w168, "OPC UA server refnum in"=w167) -> ()  [unwired: 6 in, 3 out]
        }
      }
    }
  }
  n74 = for {
    tunnel: "Array" -> [w173] mode=indexing
    tunnel: "Refnum in" -> [w171]
    tunnel: w3 -> [w170]
    n75 = Unbundle By Name(w173) -> ("name"=w169:string, "property node ID"=w172:T1)
    n76 = for {
      tunnel: w172 -> [w182]
      tunnel: w171 -> [w181]
      tunnel: w170 -> [w180] mode=indexing
      tunnel: w169 -> [w179]
      stop <- w174 stop-if-true
      n77 = Unbundle By Name(w180) -> ("Process Name"=w178:string, "User name"=w175:string)
      n78 = Concatenate Strings(w178, ":Identifier" ("string")) -> (w176:string)
      n79 = Equal?(x=w179, y=w176) -> (x = y?=w174:bool)
      n80 = case shown="True" w174 {
        tunnel: w182 -> [_ w185]
        tunnel: w181 -> [_ w184]
        tunnel: w175 -> [_ w183]
        frame False {
        }
        frame True {
          n81 = call-poly <vilib>:"Write.vi"("value"=w183, "node ID"=w185, "OPC UA server refnum in"=w184) -> ()  [unwired: 6 in, 3 out]
        }
      }
    }
  }
  n82 = for {
    tunnel: "Array" -> [w190] mode=indexing
    tunnel: "Refnum in" -> [w188]
    tunnel: w2 -> [w187]
    n83 = Unbundle By Name(w190) -> ("name"=w186:string, "property node ID"=w189:T1)
    n84 = for {
      tunnel: w189 -> [w199]
      tunnel: w188 -> [w198]
      tunnel: w187 -> [w197] mode=indexing
      tunnel: w186 -> [w196]
      stop <- w191 stop-if-true
      n85 = Unbundle By Name(w197) -> ("Process Name"=w195:string, "User name"=w192:string)
      n86 = Concatenate Strings(w195, ":Identifier" ("string")) -> (w193:string)
      n87 = Equal?(x=w196, y=w193) -> (x = y?=w191:bool)
      n88 = case shown="True" w191 {
        tunnel: w199 -> [_ w202]
        tunnel: w198 -> [_ w201]
        tunnel: w192 -> [_ w200]
        frame False {
        }
        frame True {
          n89 = call-poly <vilib>:"Write.vi"("value"=w200, "node ID"=w202, "OPC UA server refnum in"=w201) -> ()  [unwired: 6 in, 3 out]
        }
      }
    }
  }
  n90 = for {
    tunnel: "Array" -> [w207] mode=indexing
    tunnel: w1 -> [w205]
    tunnel: "Refnum in" -> [w203]
    n91 = Unbundle By Name(w207) -> ("name"=w204:string, "property node ID"=w206:T1)
    n92 = for {
      tunnel: w206 -> [w216]
      tunnel: w203 -> [w215]
      tunnel: w205 -> [w214] mode=indexing
      tunnel: w204 -> [w213]
      stop <- w208 stop-if-true
      n93 = Unbundle By Name(w214) -> ("Process Name"=w212:string, "User name"=w209:string)
      n94 = Concatenate Strings(w212, ":Identifier" ("string")) -> (w210:string)
      n95 = Equal?(x=w213, y=w210) -> (x = y?=w208:bool)
      n96 = case shown="True" w208 {
        tunnel: w216 -> [_ w219]
        tunnel: w215 -> [_ w218]
        tunnel: w209 -> [_ w217]
        frame False {
        }
        frame True {
          n97 = call-poly <vilib>:"Write.vi"("value"=w217, "node ID"=w219, "OPC UA server refnum in"=w218) -> ()  [unwired: 6 in, 3 out]
        }
      }
    }
  }
